vi "Fetch.vi"(8 "error in":errorcluster, 9 "Max Timeout":u32=10000, 10 "Fetch Type":u16(ring) items=["AC Voltage", "DC Voltage", "AC Current", "DC Current", "Real Power", "Apparent Power", "Pfactor Power", "Frequency", "Peak Current", "THD", "Current THD", "Reactive Power"], 11 "VISA resource name":refnum<visa-resource-name>) -> (0 "error out":errorcluster, 2 "Measurement":dbl format="%.3g", 3 "VISA resource name out":refnum<visa-resource-name>)   [LabVIEW 2020, in "IT-M7700.lvlib"]
doc: "Querys the actual value of the specified fetch for a desired channel.\n<b>Fetch Type</b>\n0:This command is used to read the Vrms voltage value.\n1:This command is used to read the Vdc voltage value.\n2:This command is used to read the Irms current value.\n3:This command is used to read the Idc current value.\n4:This command is used to read the active power value.\n5:This command is used to read the apparent power value.\n6:This command is used to read the power factor value.\n7:This command is used to read the frequency value.\n8:This command is used to read the maximum positive peak current reading.\n9:This command is used to read the THD.\n10:This command is used to read the current THD.\n11:This command is used to read the value of reactive power."
uses:
  <instrlib>/IT-M7700/IT-M7700.lvlib
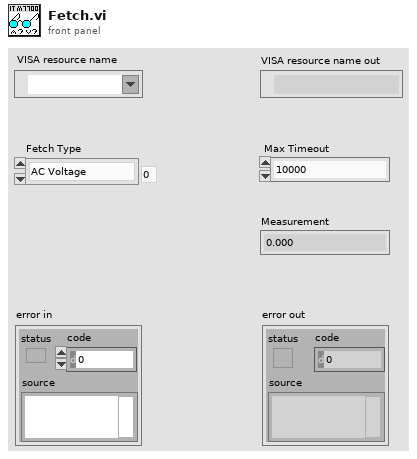
[diagram p1: front panel]
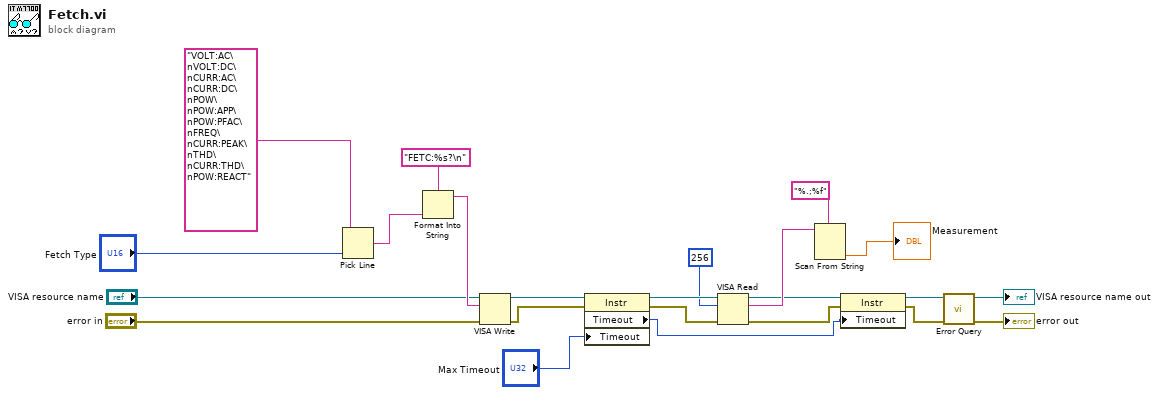
[diagram p0: block diagram]
diagram:
  n1 = Pick Line(multi-line string="VOLT:AC\nVOLT:DC\nCURR:AC\nCURR:DC\nPOW\nPOW:APP\nPOW:PFAC\nFREQ\nCURR:PEAK\nTHD\nCURR:THD\nPOW:REACT", line index="Fetch Type") -> (output string=w5:string)  [unwired: 1 in]
  n2 = Format Into String ("格式化写入字符串")(format string="FETC:%s?\n", w5) -> (resulting string=w22:string)  [unwired: 2 in, 1 out]
  n3 = VISA Write(VISA resource name="VISA resource name", write buffer=w22, error in (no error)="error in") -> (VISA resource name out=w3:refnum<visa-resource-name>, error out=w2:errorcluster)  [unwired: 1 out]
  n4 = property class="Instr"(reference=w3, error in=w2, "Timeout"="Max Timeout") -> (reference out=w17:refnum<visa-resource-name>, error out=w16:errorcluster, "Timeout"=w1:u32)
  n5 = VISA Read(VISA resource name=w17, byte count=256, error in (no error)=w16) -> (VISA resource name out=w13:refnum<visa-resource-name>, read buffer=w21:string, error out=w4:errorcluster)  [unwired: 1 out]
  n6 = Scan From String(format string="%.;%f", input string=w21) -> (output 1=→"Measurement":dbl)  [unwired: 3 in, 3 out]
  n7 = property class="Instr"(reference=w13, error in=w4, "Timeout"=w1) -> (reference out=w11:refnum<visa-resource-name>, error out=w10:errorcluster)
  n8 = call <instrlib>:"Error Query.vi"("error in"=w10, "VISA resource name"=w11) -> ("error out"=→"error out":errorcluster, "VISA resource name out"=→"VISA resource name out":refnum<visa-resource-name>)  [unwired: 6 in, 2 out]
